vi "Read Loop Times.vi"(0 "FPGA API in":refnum<class "FPGA API Concrete.lvclass">, 11 "error in (no error)":errorcluster) -> (4 "FPGA API out":refnum<class "FPGA API Concrete.lvclass">, 6 "dt(tiks) AI loop":u32, 8 "dt(tiks) DI loop":u32, 10 "dt(tiks) DO loop":u32, 14 "dt (ticks) AO Loop":u32, 15 "error out":errorcluster)   [LabVIEW 2019, in "FPGA API Concrete.lvclass"]
uses:
  FPGA API Concrete.lvclass
  FPGA API Concrete.lvclass/FPGA API Concrete.ctl
  <vilib>/Utility/error.llb/Error Cluster From Error Code.vi
  <vilib>/rvi/errors/niLvFpgaAdjustHostInterfaceError.vi
  <vilib>/rvi/interface/nirviReadWriteControl/nirviReadWriteControl.xnode
  FPGA Ref.ctl
  NiFpgaLv.dll
  <vilib>/rvi/interface/Simulation/niFpgaSimulationCallBeginRW.vi
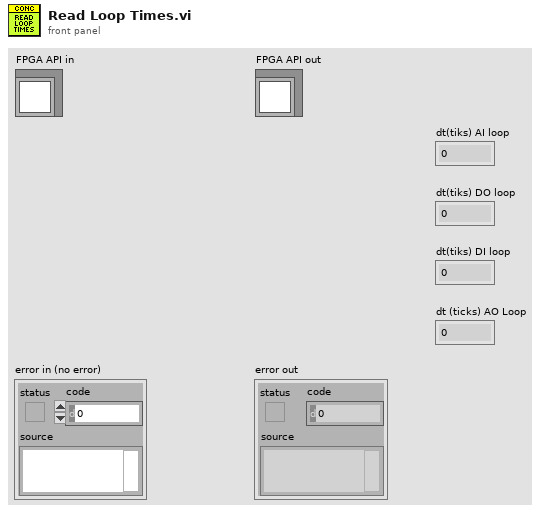
[diagram p1: front panel]
types:
  T1 = typedef "FPGA API Concrete.lvclass/FPGA Ref.ctl" = refnum<k20>
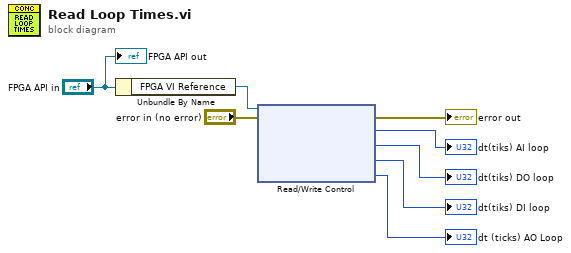
[diagram p0: block diagram]
diagram:
  n1 = Unbundle By Name("FPGA API in") -> ("FPGA VI Reference"=w3:T1)
  n2 = xnode "Read/Write Control"("FPGA VI Reference In"=w3, "error in"="error in (no error)") -> ("error out"=→"error out":errorcluster, "dt(tiks) AI loop"=→"dt(tiks) AI loop":u32, "dt(tiks) DO loop"=→"dt(tiks) DO loop":u32, "dt(tiks) DI loop"=→"dt(tiks) DI loop":u32, "dt (ticks) AO Loop"=→"dt (ticks) AO Loop":u32)  [unwired: 1 out]
  "FPGA API out" <- "FPGA API in"
